vi "VI_MAIN.vi"() -> ()   [LabVIEW 2022 SP3]
panel:
  in  "Loggin":bool
  out "Status":string
  in  "stop":bool
  in  "Password":string
  in  "User name":string
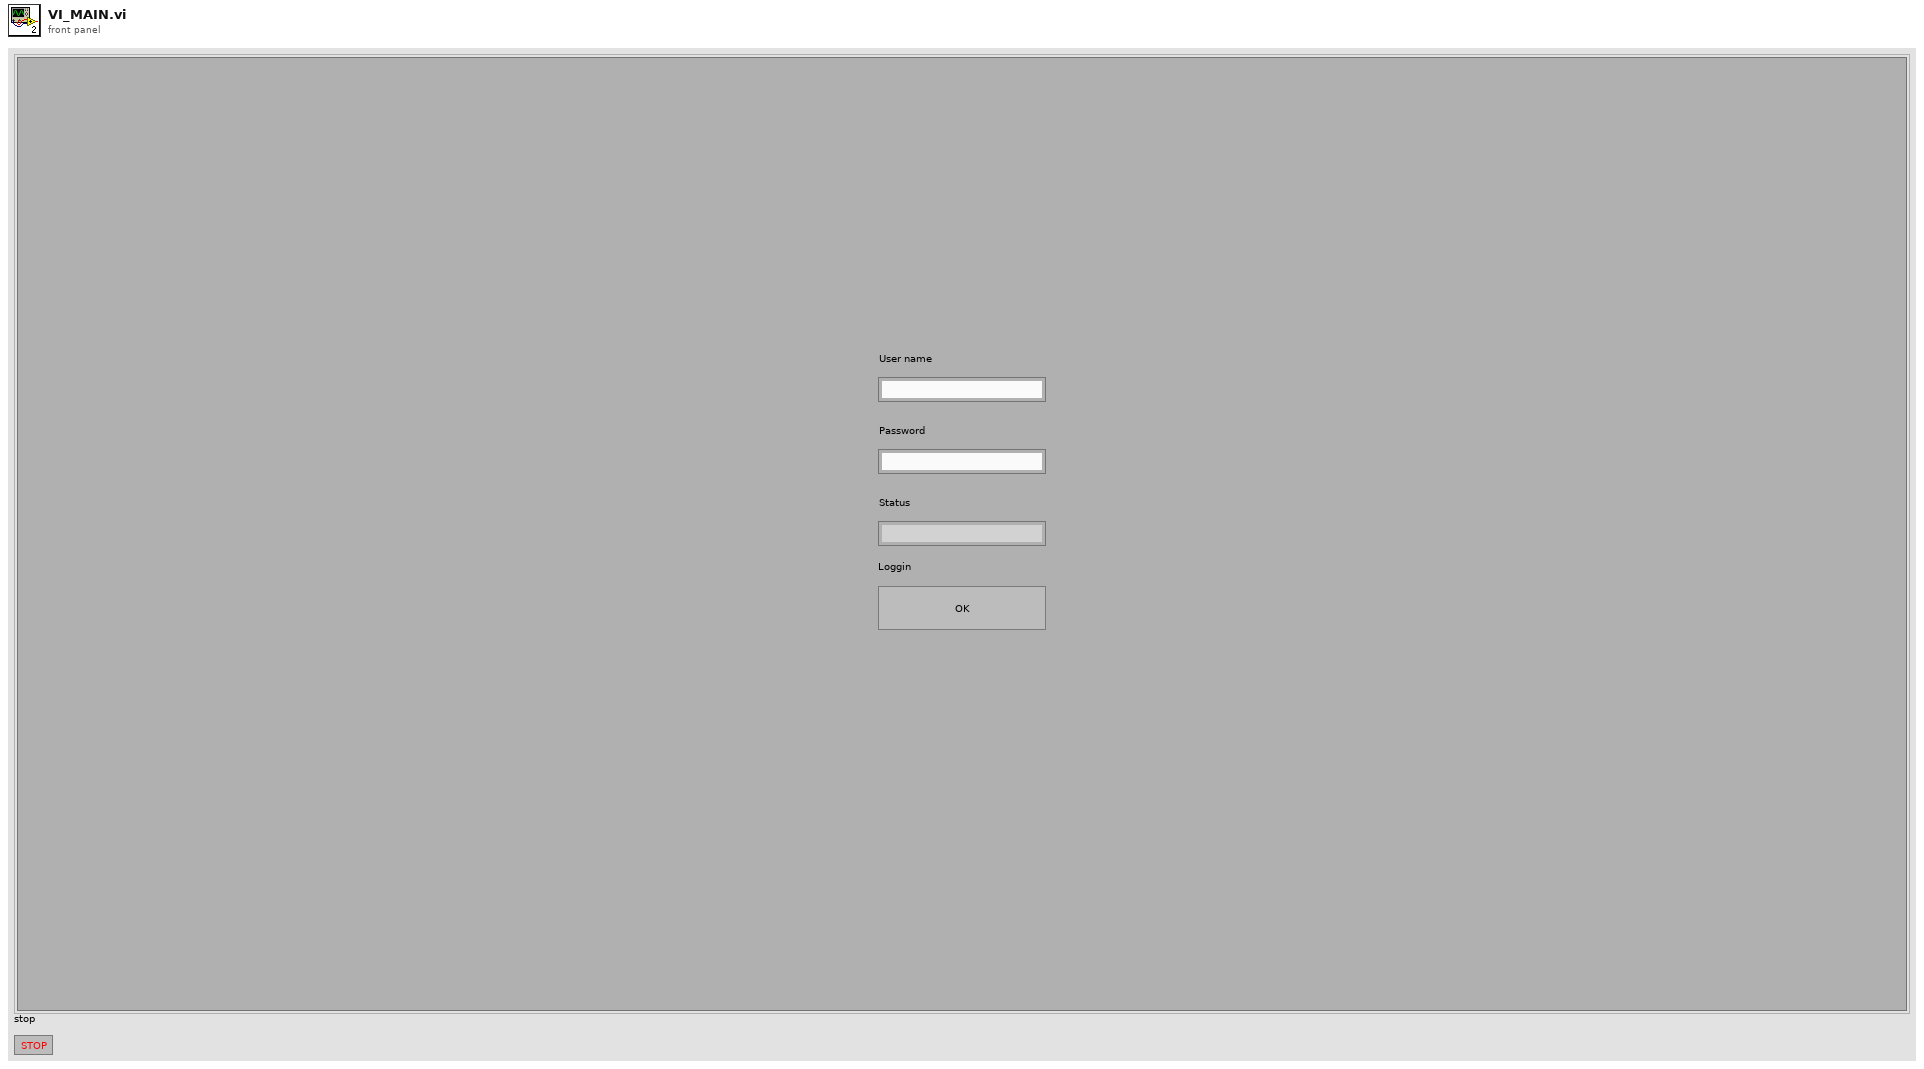
[diagram p1: front panel]
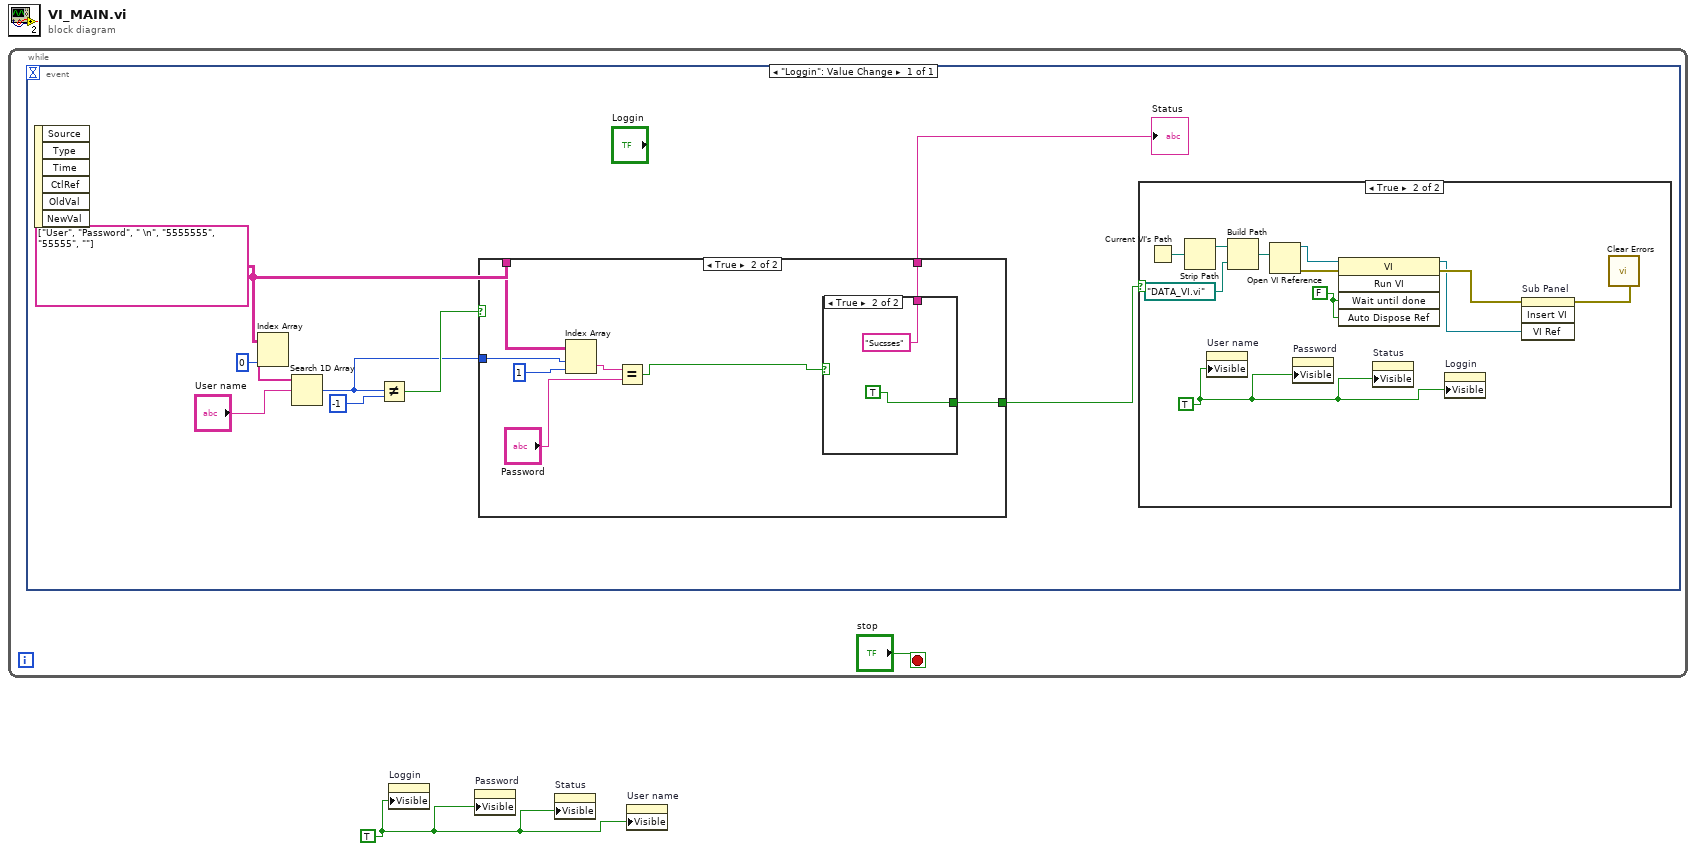
[diagram p0: block diagram]
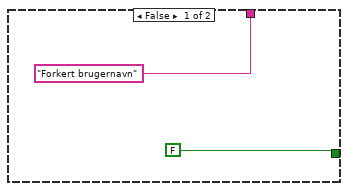
[diagram p3: hidden frame]
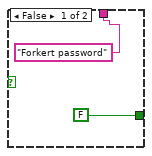
[diagram p4: hidden frame]
diagram:
  w1 = TRUE
  n1 = while {
    stop <- "stop" stop-if-true
    n2 = event shown="[0] \"Loggin\": Value Change" {
      selector: _ -> [_]
      dyn-events: _ -> [_]
      timeout: _ -> [_]
      event "Loggin": Value Change {
        w6 = string[][] [["User", "Password"], [" \n", "5555555"], ["55555", ""]]
        n3 = event-data() -> ()  [unwired: 1 in, 6 out]
        n4 = Index Array(array=w6, index (col)=0 ("disabled index (col)")) -> (element=w9:string[])  [unwired: 1 in]
        n5 = Search 1D Array(1D array=w9, element="User name") -> (index of element=w3:i32)  [unwired: 1 in]
        n6 = Not Equal?(x=w3, y=-1) -> (x != y?=w7:bool)
        n7 = case shown="True" w7 {
          tunnel: w6 -> [_ w32]
          tunnel: ["Forkert brugernavn" w30] -> w5
          tunnel: [FALSE w29] -> w4
          tunnel: w3 -> [_ w28]
          frame False {
          }
          frame True {
            n8 = Index Array(array=w32, index (row)=w28, index (col)=1 ("disabled index (col)")) -> (element=w27:string)
            n9 = Equal?(x=w27, y="Password") -> (x = y?=w25:bool)
            n10 = case shown="True" w25 {
              tunnel: ["Forkert password" "Sucsses"] -> w30
              tunnel: [FALSE TRUE] -> w29
              frame False {
              }
              frame True {
              }
            }
          }
        }
        "Status" <- w5
        n11 = case shown="True" w4 {
          frame False {
          }
          frame True {
            w12 = TRUE
            w17 = FALSE
            n12 = Current VI's Path() -> (path=w22:path)
            n13 = Strip Path(path=w22) -> (stripped path=w21:path)  [unwired: 1 out]
            n14 = property on="User name" class="Str"("Visible"=w12) -> ()  [unwired: 2 in, 2 out]
            n15 = Build Path(base path=w21, name or relative path=path "DATA_VI.vi") -> (appended path=w19:path)
            n16 = Open VI Reference(vi path=w19) -> (vi reference=w18:refnum<vi>, error out=w16:errorcluster)  [unwired: 5 in]
            n17 = property on="Password" class="Str"("Visible"=w12) -> ()  [unwired: 2 in, 2 out]
            n18 = invoke class="VI" method="Run VI"(reference=w18, error in=w16, "Wait until done"=w17, "Auto Dispose Ref"=w17) -> (reference out=w14:refnum<vi>, error out=w15:errorcluster)  [unwired: 1 in, 3 out]
            n19 = property on="Status" class="Str"("Visible"=w12) -> ()  [unwired: 2 in, 2 out]
            n20 = property on="Loggin" class="Bool"("Visible"=w12) -> ()  [unwired: 2 in, 2 out]
            n21 = invoke on="Sub Panel" class="SubPnl" method="Insert VI"(error in=w15, "VI Ref"=w14) -> (error out=w13:errorcluster)  [unwired: 2 in, 3 out]
            n22 = call <vilib>:"Clear Errors.vi"("error in (no error)"=w13) -> ()  [unwired: 5 in, 2 out]
          }
        }
      }
    }
  }
  n23 = property on="Loggin" class="Bool"("Visible"=w1) -> ()  [unwired: 2 in, 2 out]
  n24 = property on="Password" class="Str"("Visible"=w1) -> ()  [unwired: 2 in, 2 out]
  n25 = property on="Status" class="Str"("Visible"=w1) -> ()  [unwired: 2 in, 2 out]
  n26 = property on="User name" class="Str"("Visible"=w1) -> ()  [unwired: 2 in, 2 out]
